vi "Poll Pumps.vi"(8 "error in (no error)":errorcluster, 11 "App Data":T1={"Pump Station Controls"={"Lag Pump"=enum."OFF", "Lead Pump"=enum."OFF", "ALARM"=0.0, "LAG"=0.0, "LEAD"=0.0, "STOP"=0.0}, "Pump Indicators"={"Pump Water Level"=0.0, "ALARM"=FALSE, "LAG"=FALSE, "LEAD"=FALSE, "STOP"=FALSE, "PUMP 1 STATE"=FALSE, "PUMP 2 STATE"=FALSE}, "Alarm"=refnum, "Lag Start Time"=timestamp(0 s since 1904-01-01), "Lead Start Time"=timestamp(0 s since 1904-01-01), "Main Q"=refnum} {"Pump Indicators"."Pump Water Level" scale=0.0..4.0}) -> (0 "error out":errorcluster, 3 "App Data Out":T1={"Pump Station Controls"={"Lag Pump"=enum."OFF", "Lead Pump"=enum."OFF", "ALARM"=0.0, "LAG"=0.0, "LEAD"=0.0, "STOP"=0.0}, "Pump Indicators"={"Pump Water Level"=0.0, "ALARM"=FALSE, "LAG"=FALSE, "LEAD"=FALSE, "STOP"=FALSE, "PUMP 1 STATE"=FALSE, "PUMP 2 STATE"=FALSE}, "Alarm"=refnum, "Lag Start Time"=timestamp(0 s since 1904-01-01), "Lead Start Time"=timestamp(0 s since 1904-01-01), "Main Q"=refnum} {"Pump Indicators"."Pump Water Level" scale=0.0..4.0})   [LabVIEW 2024]
uses:
  App Data.ctl
  Pump Controls.ctl
  Pump Switch.ctl
  Pump Indicators.ctl
  Q Info.ctl
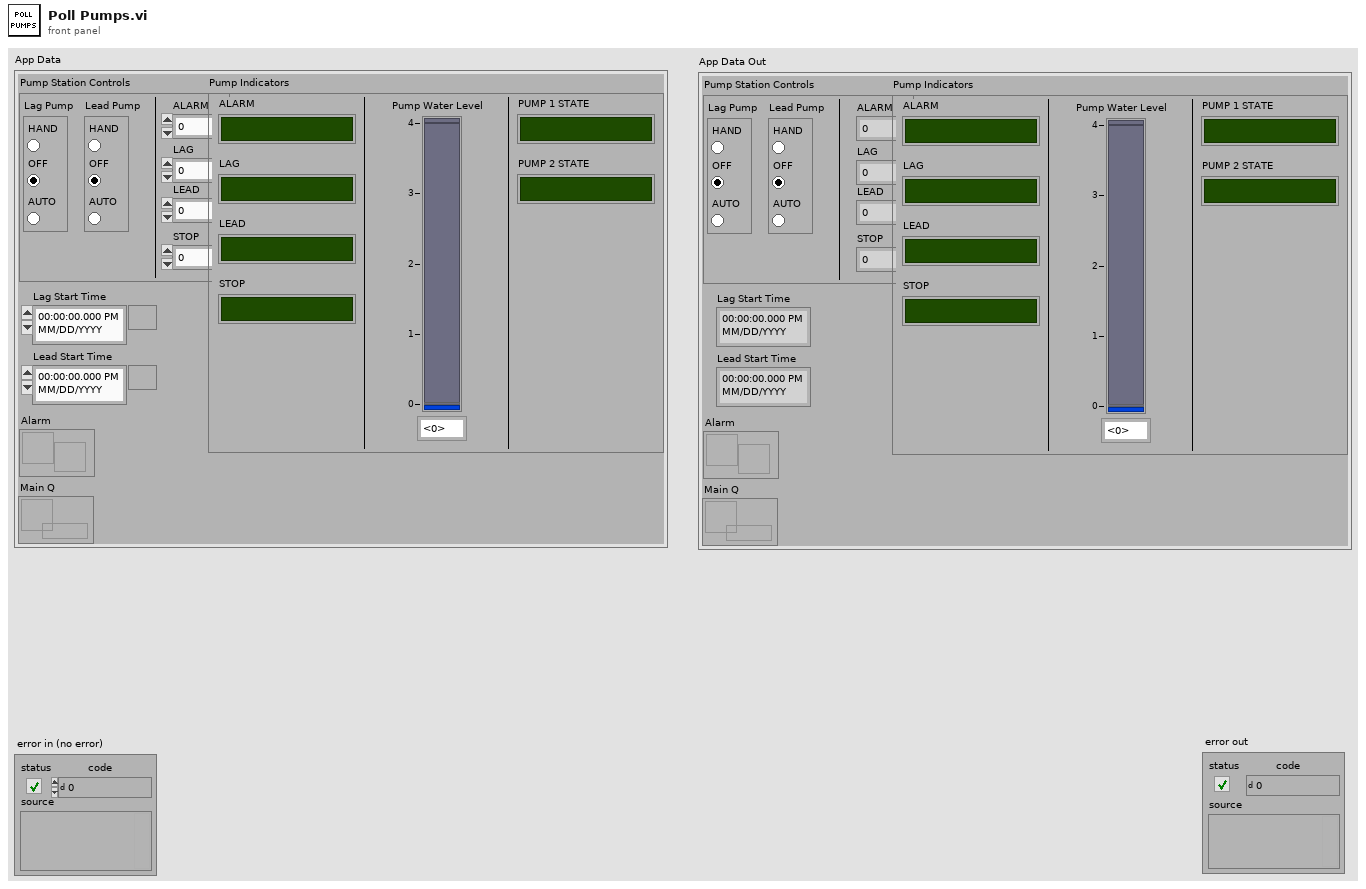
[diagram p1: front panel]
types:
  T1 = typedef "App Data.ctl" = cluster{"Pump Station Controls":T2, "Pump Indicators":T4, "Alarm":refnum<notifier>, "Lag Start Time":timestamp, "Lead Start Time":timestamp, "Main Q":refnum<queue>}
  T2 = typedef "Pump Controls.ctl" = cluster{"Lag Pump":T3, "Lead Pump":T3, "ALARM":dbl, "LAG":dbl, "LEAD":dbl, "STOP":dbl}
  T3 = typedef "Pump Switch.ctl" = enum32{"HAND", "OFF", "AUTO"}
  T4 = typedef "Pump Indicators.ctl" = cluster{"Pump Water Level":dbl, "ALARM":bool, "LAG":bool, "LEAD":bool, "STOP":bool, "PUMP 1 STATE":bool, "PUMP 2 STATE":bool}
  T5 = typedef "Q Info.ctl" = cluster{"State":string, "Data":variant}
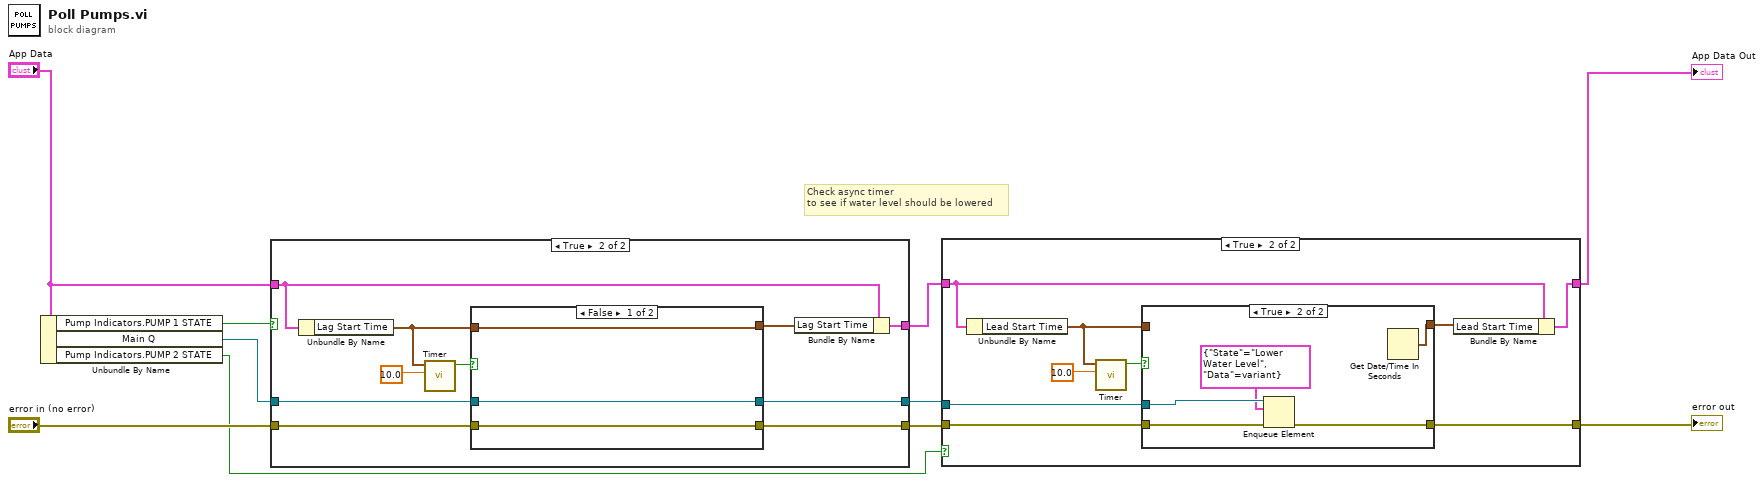
[diagram p0: block diagram]
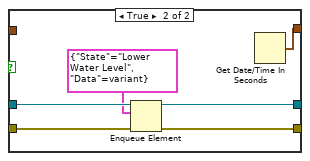
[diagram p5: hidden frame]
diagram:
  # "Check async timer \nto see if water level should be lowered"
  n1 = Unbundle By Name("App Data") -> ("Pump Indicators.PUMP 1 STATE"=w10:bool, "Main Q"=w7:refnum<queue>, "Pump Indicators.PUMP 2 STATE"=w1:bool)
  n2 = case shown="True" w10 {
    tunnel: "App Data" -> [w13 w18]
    tunnel: "error in (no error)" -> [w11 w20]
    tunnel: w7 -> [w12 w19]
    tunnel: [w13 w16] -> w6
    tunnel: [w12 w15] -> w5
    tunnel: [w11 w14] -> w4
    frame False {
    }
    frame True {
      n3 = Unbundle By Name(w18) -> ("Lag Start Time"=w21:timestamp)
      n4 = call "Timer.vi"("Time Target"=10.0, "Last iteration Time"=w21) -> ("Time Elapsed?"=w22:bool)  [unwired: 9 in]
      n5 = case shown="False" w22 {
        tunnel: w21 -> [w26 _]
        tunnel: w20 -> [w24 w32]
        tunnel: w19 -> [w25 w31]
        tunnel: [w26 w29] -> w17
        tunnel: [w25 w28] -> w15
        tunnel: [w24 w27] -> w14
        frame False {
        }
        frame True {
          n6 = Enqueue Element(queue=w31, element=T5 {"State"="Lower Water Level", "Data"=variant}, error in (no error)=w32) -> (queue out=w28:refnum<queue>, error out=w27:errorcluster)  [unwired: 1 in, 1 out]
          n7 = Get Date/Time In Seconds() -> (seconds since 1Jan1904=w29:timestamp)
        }
      }
      n8 = Bundle By Name(cluster=w18, "Lag Start Time"=w17) -> (w16:T1)
    }
  }
  n9 = case shown="True" w1 {
    tunnel: w6 -> [w33 w38]
    tunnel: w4 -> [w34 w40]
    tunnel: w5 -> [_ w39]
    tunnel: [w34 w36] -> w3
    tunnel: [w33 w35] -> w2
    frame False {
    }
    frame True {
      n10 = Unbundle By Name(w38) -> ("Lead Start Time"=w41:timestamp)
      n11 = call "Timer.vi"("Time Target"=10.0, "Last iteration Time"=w41) -> ("Time Elapsed?"=w42:bool)  [unwired: 9 in]
      n12 = case shown="True" w42 {
        tunnel: w41 -> [w45 _]
        tunnel: w40 -> [w44 w50]
        tunnel: w39 -> [_ w49]
        tunnel: [w45 w47] -> w37
        tunnel: [w44 w46] -> w36
        frame False {
        }
        frame True {
          n13 = Enqueue Element(queue=w49, element=T5 {"State"="Lower Water Level", "Data"=variant}, error in (no error)=w50) -> (error out=w46:errorcluster)  [unwired: 1 in, 2 out]
          n14 = Get Date/Time In Seconds() -> (seconds since 1Jan1904=w47:timestamp)
        }
      }
      n15 = Bundle By Name(cluster=w38, "Lead Start Time"=w37) -> (w35:T1)
    }
  }
  "App Data Out" <- w2
  "error out" <- w3
